vi "Reset FGV.vi"(11 "Get? (T)":bool=TRUE) -> (3 "Reset?":bool)   [LabVIEW 2017]
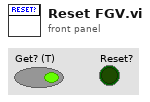
[diagram p1: front panel]
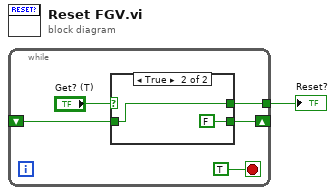
[diagram p0: block diagram]
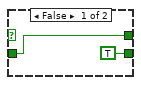
[diagram p2: hidden frame]
diagram:
  n1 = while {
    shift-right: [w4] -> _
    shift-left: _ -> [w3]
    tunnel: [w2] -> w1
    stop <- TRUE stop-if-true
    n2 = case shown="True" "Get? (T)" {
      tunnel: [TRUE FALSE] -> w4
      tunnel: w3 -> [w7 w9]
      tunnel: [w7 w9] -> w2
      frame False {
      }
      frame True {
      }
    }
  }
  "Reset?" <- w1
